vi "FindRealClassTypeObject.vi"(0 "flattened remote ref":string, 5 "error in (no error)":errorcluster) -> (12 "G#DebugServer ref":refnum<class "G#Object.lvclass">, 14 "real ibject ref":refnum<class "G#Object.lvclass">, 15 "not found?":bool, 16 "in host memory?":bool, 19 "error out":errorcluster)   [LabVIEW 2020, in "G#DebugServer.lvclass"]
doc: "Finds the real class type object."
uses:
  G#DebugServer.lvclass
  G#Object/G#Object.lvclass
  C:/ProjectGSharpDevelopment/gsharp/VIPM/Files/vi.lib/addons/_AddQ/G#Object/G#Object.lvclass
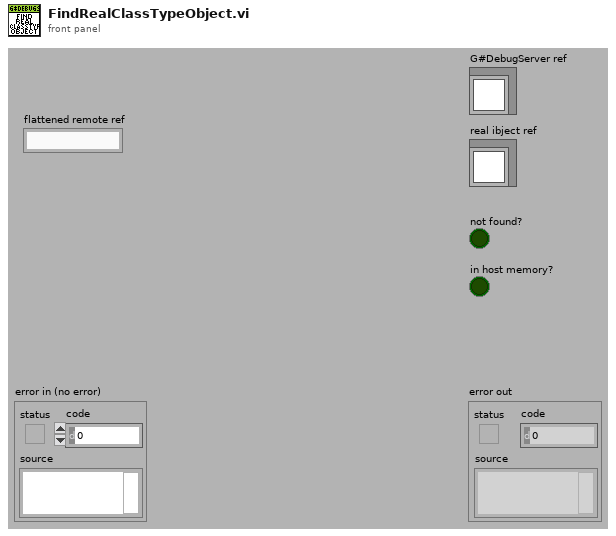
[diagram p1: front panel]
types:
  T1 = cluster{bool, "G#Object reference in":refnum<class "G#Object.lvclass">}
  T2 = typedef "G#Object.lvclass/G#Object_ClassInfoType.ctl" = cluster{"ClassName":string, "ObjectInfo":T3[], "ObjectRefs":refnum<class "G#Object.lvclass">[], "TypeRef":refnum<class "G#Object.lvclass">}
  T3 = typedef "G#Object.lvclass/G#Object_ObjectInfoType.ctl" = cluster{"ObjectName":string, "ObjectID":u32, "Users":i32, "Counter":bool, "AttributeRefs":u32[], "FullClassName":string, "ClassName":string, "CreateMethod":T4, "GenericDestructorExists":bool, "Owner":string}
  T4 = typedef "G#Object.lvclass/G#Object_CreateMethod.ctl" = enum16{"Create", "Create or look up existing", "Look up existing"}
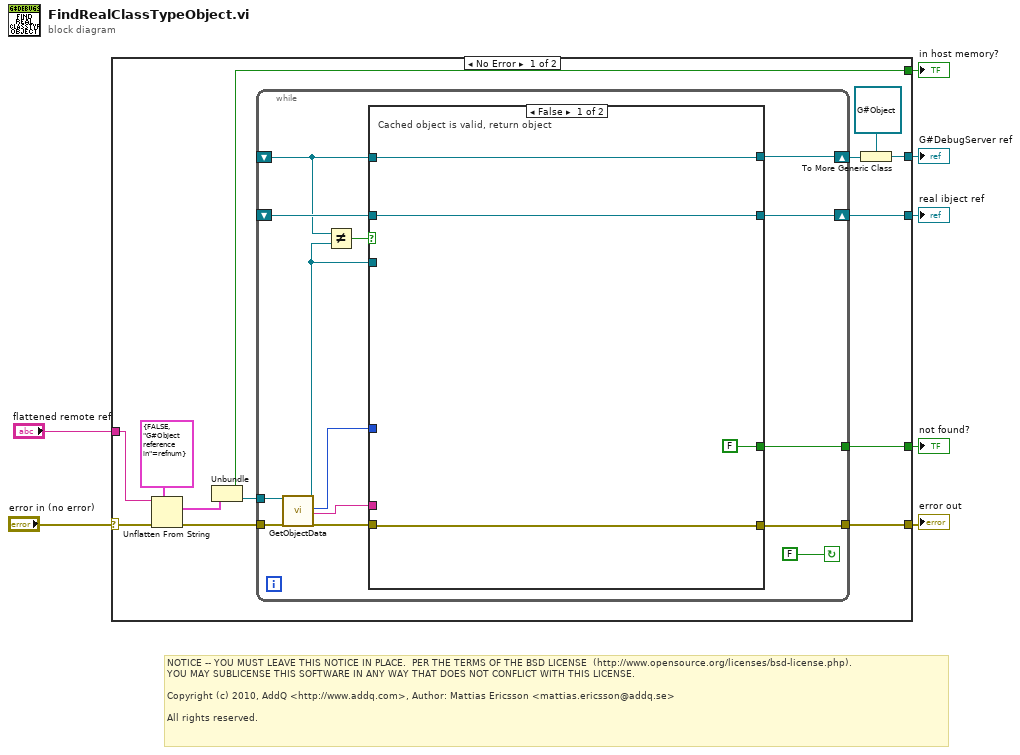
[diagram p0: block diagram]
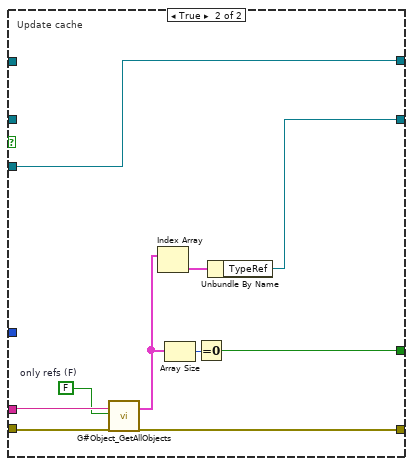
[diagram p2: hidden frame]
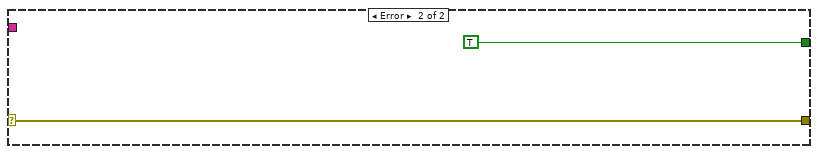
[diagram p3: hidden frame]
diagram:
  # "NOTICE -- YOU MUST LEAVE THIS NOTICE IN PLACE.  PER THE TERMS OF THE BSD LICENSE  (http://www.opensource.org/licenses/bsd-license.php).\nYOU MAY SUBLICENSE THIS SOFTWARE IN ANY WAY THAT DOES NOT CONFLICT WITH THIS LICENSE.\n\nCopyright (c) 2010, AddQ <http://www.addq.com>, Author: Mattias Ericsson <mattias.ericsson@addq.se>\n\nAll rights reserved."
  n1 = case shown="No Error" "error in (no error)" {
    selector: "error in (no error)" -> [w17 w50]
    tunnel: [w20 w50] -> w6
    tunnel: [w19 TRUE] -> w5
    tunnel: [w18 _] -> w4
    tunnel: "flattened remote ref" -> [w12 _]
    tunnel: [w14 _] -> w2
    tunnel: [w8 _] -> w1
    frame No Error {
      n2 = Unflatten From String(type=T1 {FALSE, "G#Object reference in"=refnum}, binary string=w12, error in (no error)=w17) -> (value=w9:T1, error out=w16:errorcluster)  [unwired: 2 in, 1 out]
      n3 = Unbundle(w9) -> (w8:bool, "G#Object reference in"=w10:refnum<class "G#Object.lvclass">)
      n4 = while {
        tunnel: w16 -> [w34]
        tunnel: [w25] -> w20
        shift-right: [w31] -> w13
        shift-left: _ -> [w22]
        shift-right: [w23] -> w18
        shift-left: _ -> [w26]
        tunnel: [w24] -> w19
        tunnel: w10 -> [w21]
        stop <- FALSE continue-if-true
        n5 = call "GetObjectData.vi"("remote ref"=w21, "error in (no error)"=w34) -> ("G#DebugServer reference out"=w33:refnum<class "G#DebugServer.lvclass">, "ObjectID"=w29:u32, "FullClassName"=w28:string, "error out"=w27:errorcluster)  [unwired: 13 in, 1 out]
        n6 = Not Equal?(x=w22, y=w33) -> (x != y?=w32:bool)
        n7 = case shown="False" w32 {
          tunnel: w33 -> [_ w48]
          tunnel: [w38 w48] -> w31
          tunnel: w22 -> [w38 _]
          tunnel: w29 -> [_ _]
          tunnel: w28 -> [_ w46]
          tunnel: w27 -> [w36 w47]
          tunnel: w26 -> [w37 _]
          tunnel: [w36 w43] -> w25
          tunnel: [FALSE w40] -> w24
          tunnel: [w37 w39] -> w23
          frame False {
            # "Cached object is valid, return object"
          }
          frame True {
            w45 = FALSE  # only refs (F)
            # "Update cache"
            n8 = call "G#Object_GetAllObjects.vi"("full class name (\"\")"=w46, "only refs (F)"=w45, "error in (no error)"=w47) -> ("class information"=w42:T2[], "error out"=w43:errorcluster)  [unwired: 13 in, 2 out]
            n9 = Index Array(array=w42) -> (element=w44:T2)  [unwired: 1 in]
            n10 = Array Size(array=w42) -> (size(s)=w41:i32)
            n11 = Equal To 0?(x=w41) -> (x = 0?=w40:bool)
            n12 = Unbundle By Name(w44) -> ("TypeRef"=w39:refnum<class "G#Object.lvclass">)
          }
        }
      }
      n13 = To More Generic Class(target class=refnum<class "G#Object.lvclass"> refnum ("G#Object reference in"), reference=w13) -> (generic class reference=w14:refnum<class "G#Object.lvclass">)
    }
    frame Error {
    }
  }
  "error out" <- w6
  "not found?" <- w5
  "real ibject ref" <- w4
  "G#DebugServer ref" <- w2
  "in host memory?" <- w1
